vi "LVObject to JSON.vi"(5 "enable LabVIEW extensions? (T)":bool=TRUE, 6 "Pretty Print?":bool, 7 "Class 1 in":refnum<class "Serializer-Palette.lvclass">, 8 "error in":errorcluster, 10 "Object":refnum<class>) -> (0 "error out":errorcluster, 2 "<JSON>Object":string)   [LabVIEW 2021, in "TSC Material Theme.lvlib" / "Serializer-Palette.lvclass"]
doc: "Convert Object of a LabVIEW Class to a JSON representation."
uses:
  Serializer-Palette.lvclass
  Material-Palette/Material-Palette.lvclass
  Material-Palette/Material-Palette.lvclass/Material-Palette.ctl
  <vilib>/JDP Science/JSONtext/JSONtext.lvlib
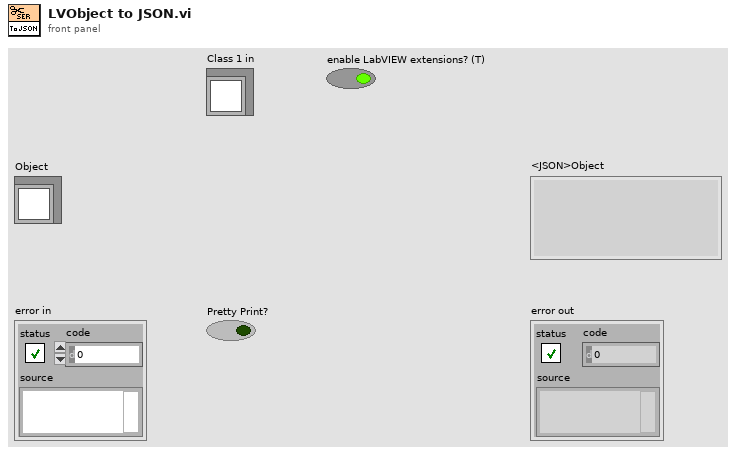
[diagram p1: front panel]
types:
  T1 = typedef "TSC Material Theme.lvlib/material json palette--cluster.ctl" = cluster{"0":string, "5":string, "10":string, "15":string, "20":string, "25":string, "30":string, "35":string, "40":string, "50":string, "60":string, "70":string, "80":string, "90":string, "95":string, "98":string, "99":string, "100":string}
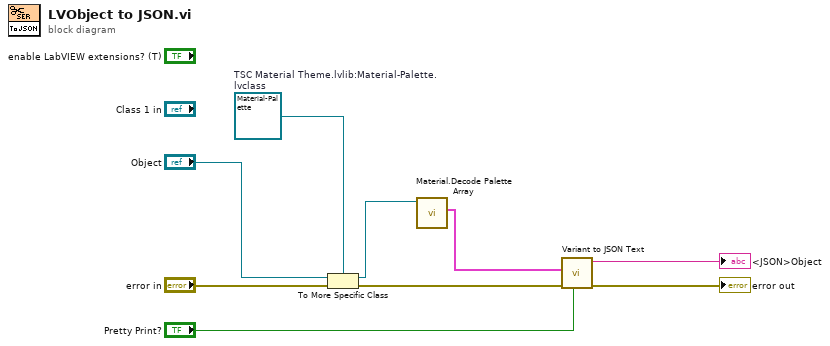
[diagram p0: block diagram]
diagram:
  w5 = refnum<class "Material-Palette.lvclass"> refnum  # TSC Material Theme.lvlib:Material-Palette.lvclass
  n1 = To More Specific Class(target class=w5, reference="Object", error in="error in") -> (specific class reference=w4:refnum<class "Material-Palette.lvclass">, error out=w8:errorcluster)
  n2 = call "Material.Decode Palette Array.vi"("Palettes"=w4) -> ("palette"=w3:T1)  [unwired: 10 in]
  n3 = call <vilib>:"Variant to JSON Text.vi"("Pretty Print?"="Pretty Print?", "error in (no error)"=w8, "Variant"=w3) -> ("error out"=→"error out":errorcluster, "<JSON>"=→"<JSON>Object":string)  [unwired: 6 in, 1 out]
